vi "RS485.vi"() -> ()   [LabVIEW 2018]
uses:
  <vilib>/Instr/_visa.llb/VISA Configure Serial Port (Instr).vi
panel:
  in  "baud rate":u32=19200
  out "버퍼 수신(16진수)":u8[](array[numeric]) format="%02x"
  out "버퍼 수신(10진수)":u8[](array[numeric]) format="%02d"
  out "송신 시간":string
  out "to 10진수":u8[](array[numeric])
  in  "from 16진수":u8[](array[numeric]) format="%02x"
  out "버퍼 송신(10진수)":u8[](array[numeric]) format="%02d"
  out "버퍼 송신(16진수)":u8[](array[numeric]) format="%02x"
  in  "from 10진수":u8[](array[numeric])
  out "to 16진수":u8[](array[numeric]) format="%02x"
  in  "버퍼 송신":string
  in  "정지":bool
  in  "command":u8[](array[numeric])=[183, 172, 2, 130, 2]
  out "수신 시간":string
  in  "VISA resource name":refnum<visa-resource-name>
  out "버퍼 수신":string
  in  "Write":bool
  # "RMID"
  # "TMID"
  # "ID"
  # "PID"
  # "Data#"
  # "Data"
  # "RMID"
  # "TMID"
  # "ID"
  # "PID"
  # "Data#"
  # "Data"
  # "Read 183 172 1 4 1 133 chksum"
  # "RMID"
  # "TMID"
  # "ID"
  # "PID"
  # "Data#"
  # "Data"
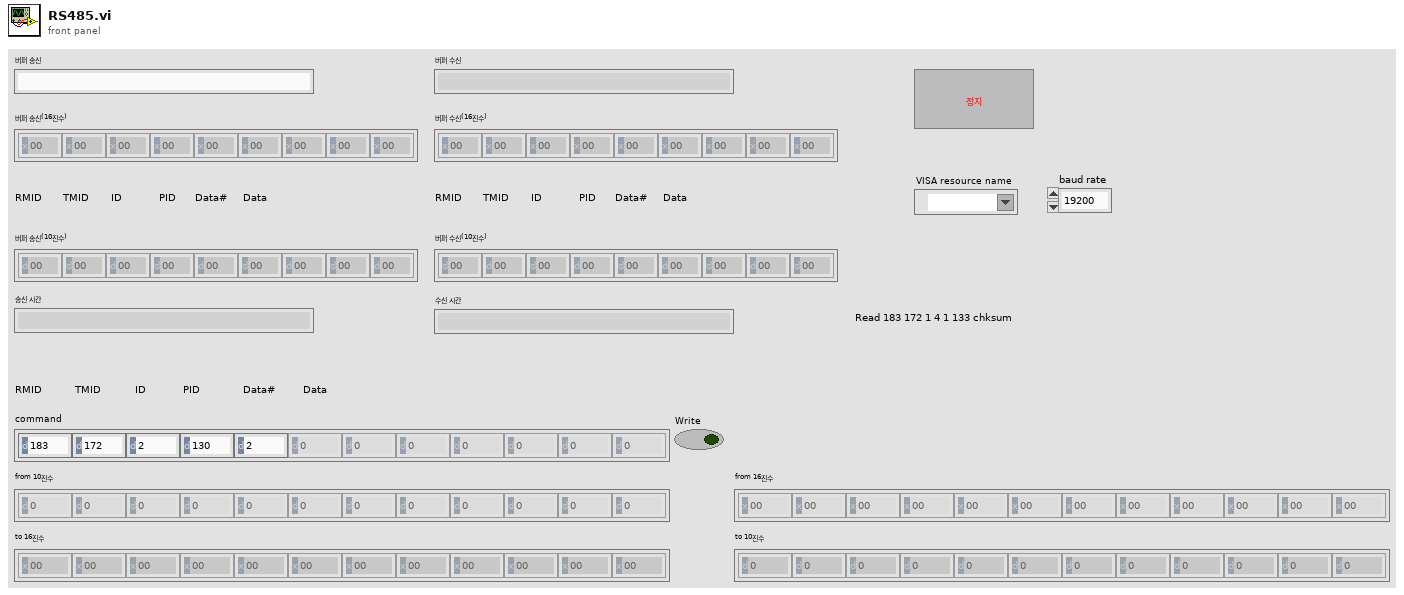
[diagram p1: front panel]
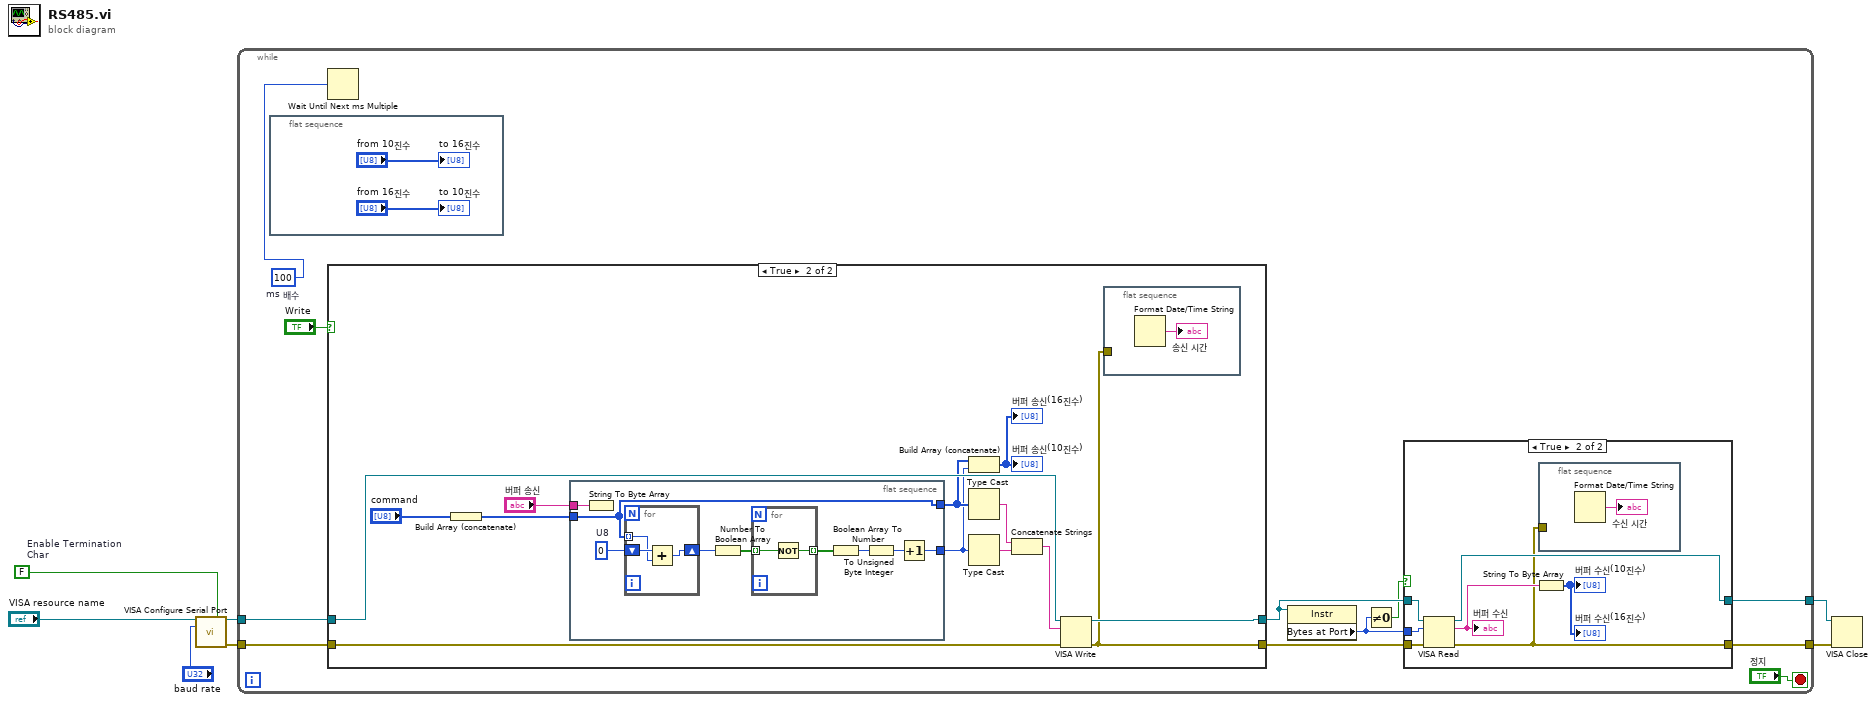
[diagram p0: block diagram]
diagram:
  w3 = FALSE  # Enable Termination Char
  n1 = call-poly "VISA Configure Serial Port"("VISA resource name"="VISA resource name", "Enable Termination\nChar (T)"=w3, "baud rate (9600)"="baud rate") -> ("VISA resource name out"=w7:refnum<visa-resource-name>, "error out"=w1:errorcluster)  [unwired: 11 in]
  n2 = while {
    tunnel: w7 -> [w18]
    tunnel: [w17] -> w6
    tunnel: [w14] -> w2
    tunnel: w1 -> [w12]
    stop <- "정지" stop-if-true
    w11 = u32 100  # ms 배수
    n3 = flat-sequence {
      frame #0 {
        "to 16진수" <- "from 10진수"
        "to 10진수" <- "from 16진수"
      }
    }
    n4 = Wait Until Next ms Multiple(millisecond multiple=w11) -> ()  [unwired: 1 out]
    n5 = case shown="True" "Write" {
      tunnel: w18 -> [w32 w45]
      tunnel: [w32 w44] -> w15
      tunnel: [w31 w33] -> w13
      tunnel: w12 -> [w31 w43]
      frame False {
      }
      frame True {
        n6 = Build Array (concatenate)("command") -> (w39:u8[])
        n7 = flat-sequence {
          tunnel: [w49] -> w35
          tunnel: w39 -> [w47]
          tunnel: [w47] -> w36
          tunnel: "버퍼 송신" -> [w48]
          frame #0 {
            w55 = u8 0  # U8
            n8 = String To Byte Array(string=w48) -> ()  [unwired: 1 out]
            n9 = for {
              tunnel: w47 -> [w59] mode=indexing
              shift-right: [w58] -> w54
              shift-left: w55 -> [w60]
              n10 = Add(x=w60, y=w59) -> (x+y=w58:u8)
            }
            n11 = Number To Boolean Array(number=w54) -> (Boolean array=w53:bool[])
            n12 = for {
              tunnel: w53 -> [w57] mode=indexing
              tunnel: [w56] -> w52 mode=indexing
              n13 = Not(x=w57) -> (.not. x?=w56:bool)
            }
            n14 = Boolean Array To Number(Boolean array=w52) -> (number=w51:u32)
            n15 = To Unsigned Byte Integer(number=w51) -> (unsigned 8bit integer=w50:u8)
            n16 = Increment(x=w50) -> (x+1=w49:u8)
          }
        }
        n17 = Build Array (concatenate)(w36, w35) -> (→"버퍼 송신(16진수)" →"버퍼 송신(10진수)":u8[])
        n18 = Type Cast(x=w36) -> (*(type *) &x=w38:string)  [unwired: 1 in]
        n19 = Type Cast(x=w35) -> (*(type *) &x=w42:string)  [unwired: 1 in]
        n20 = Concatenate Strings(w38, w42) -> (w41:string)
        n21 = VISA Write(VISA resource name=w45, write buffer=w41, error in (no error)=w43) -> (VISA resource name out=w44:refnum<visa-resource-name>, error out=w33:errorcluster)  [unwired: 1 out]
        n22 = flat-sequence {
          tunnel: w33 -> [_]
          frame #0 {
            n23 = Format Date/Time String() -> (date/time string=→"송신 시간":string)  [unwired: 3 in]
          }
        }
      }
    }
    n24 = property class="Instr"(reference=w15) -> ("Bytes at Port"=w8:u32)  [unwired: 1 in, 2 out]
    n25 = Not Equal To 0?(x=w8) -> (x != 0?=w9:bool)
    n26 = case shown="True" w9 {
      tunnel: w15 -> [w22 w29]
      tunnel: [w22 w28] -> w17
      tunnel: [w21 w24] -> w14
      tunnel: w8 -> [_ w27]
      tunnel: w13 -> [w21 w26]
      frame False {
      }
      frame True {
        n27 = VISA Read(VISA resource name=w29, byte count=w27, error in (no error)=w26) -> (VISA resource name out=w28:refnum<visa-resource-name>, read buffer=w25:string, error out=w24:errorcluster)  [unwired: 1 out]
        "버퍼 수신" <- w25
        n28 = String To Byte Array(string=w25) -> (unsigned byte array=→"버퍼 수신(16진수)" →"버퍼 수신(10진수)":u8[])
        n29 = flat-sequence {
          tunnel: w24 -> [_]
          frame #0 {
            n30 = Format Date/Time String() -> (date/time string=→"수신 시간":string)  [unwired: 3 in]
          }
        }
      }
    }
  }
  n31 = VISA Close(VISA resource name=w6, error in (no error)=w2) -> ()  [unwired: 1 out]
